vi "test_MultipleSessionsReserved_CallCreateSession_NothingAddedToConnectionMap.vi"(8 "error in":errorcluster) -> (0 "error out":errorcluster, 2 "result":string, 3 "pass":bool)   [LabVIEW 2020, in "MeasurementServerTests.lvlib"]
uses:
  MeasurementServerTests.lvlib
  Runtime/MeasurementLink Session Management/Session Reservation/Connection with Session.ctl
  Runtime/MeasurementLink Session Management/Session Reservation/Connection.ctl
  1a7c149c-48bc-4238-8756-811e337da54d.vi
  a956f7ee-c7e9-4639-884c-f4265dae6ecf.vi
  da202071-85ff-4e27-b7cd-0a9c854c86e4.vi
  da202071-85ff-4e27-b7cd-0a9c854c86e4.vi/7fd45821-cfd3-468e-85e7-fb0eb05eda95.vi
  Helpers/Fake Instrument/Fake Instrument.lvclass
  C:/dev/measurementlink-labview/Source/Runtime/MeasurementLink Instrument/IInstrument/IInstrument.lvclass
  Runtime/MeasurementLink Measurement Server/Helpers/Error Strings Global Internal.vi
  Runtime/MeasurementLink Session Management/Session Reservation/Create Sessions Dispatcher.vi
  Runtime/MeasurementLink Session Management/Session Reservation/Get Connections Dispatcher.vi
  Runtime/MeasurementLink Session Management/Session Reservation/Session Reservation.lvclass
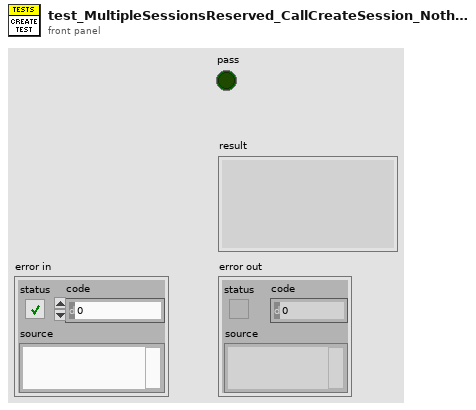
[diagram p1: front panel]
types:
  T1 = typedef "MeasurementLink Session Management.lvlib/Session Reservation.lvclass/Connection with Session.ctl" = cluster{"connection":T2, "session":variant}
  T2 = typedef "MeasurementLink Session Management.lvlib/Session Reservation.lvclass/Connection.ctl" = cluster{"pin or relay name":string, "site":i32, "instrument type id":string, "channel":string}
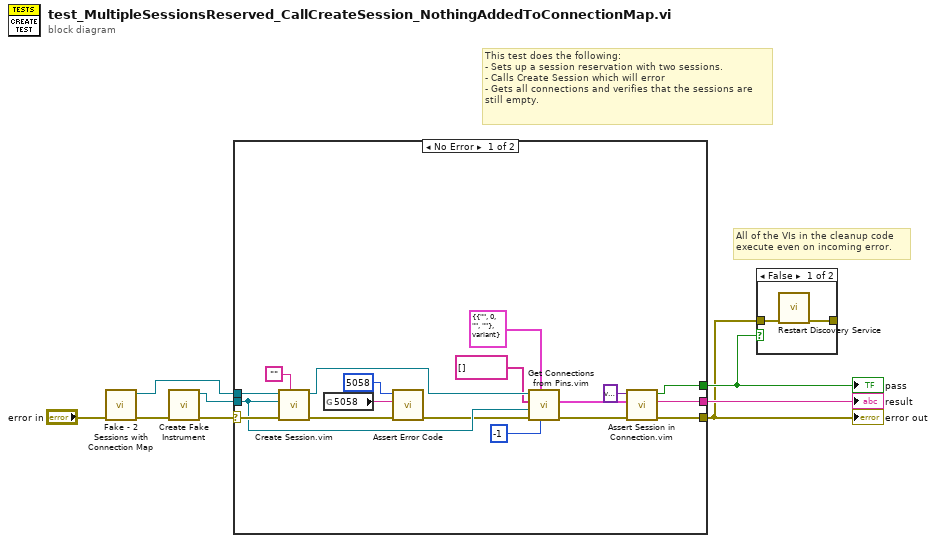
[diagram p0: block diagram]
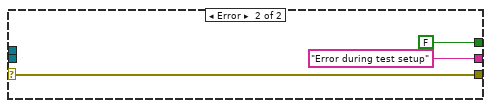
[diagram p2: hidden frame]
diagram:
  # "All of the VIs in the cleanup code\nexecute even on incoming error."
  # "This test does the following:\n- Sets up a session reservation with two sessions.\n- Calls Create Session which will error \n- Gets all connections and verifies that the sessions are\nstill empty."
  n1 = call "Fake - 2 Sessions with Connection Map.vi"("error in"="error in") -> ("error out"=w2:errorcluster, "session reservation out"=w1:refnum<class "Session Reservation.lvclass">)  [unwired: 9 in]
  n2 = call "Create Fake Instrument.vi"("error in"=w2) -> ("error out"=w5:errorcluster, "fake instrument out"=w4:refnum<class "Fake Instrument.lvclass">)  [unwired: 9 in]
  n3 = case shown="No Error" w5 {
    selector: w5 -> [w24 w26]
    tunnel: [w17 w26] -> w6
    tunnel: [w10 FALSE] -> w7
    tunnel: [w9 "Error during test setup" ("f")] -> w8
    tunnel: w4 -> [w20 _]
    tunnel: w1 -> [w25 _]
    frame No Error {
      n4 = call "Create Session.vim"("session type"="", "error in"=w24, "instrument"=w20, "session reservation in"=w25) -> ("error out"=w16:errorcluster, "session reservation out"=w22:refnum<class "Session Reservation.lvclass">)  [unwired: 4 in, 2 out]
      n5 = global read "Error Strings Global Internal.vi" "5058"() -> (w14:string)
      n6 = call "Assert Error Code.vi"("error in"=w16, "expected error description"=w14, "expected error code"=5058) -> ("error out"=w15:errorcluster)  [unwired: 6 in, 2 out]
      n7 = call "Get Connections from Pins.vim"("site"=-1, "connection type"=T1 {"connection"={"pin or relay name"="", "site"=0, "instrument type id"="", "channel"=""}, "session"=variant}, "error in"=w15, "instrument"=w20, "pin or relay names"=string[] [], "session reservation in"=w22) -> ("error out"=w17:errorcluster, "connections"=w12:T1[])  [unwired: 3 in, 1 out]
      n8 = call "Assert Session in Connection.vim"("actual connections"=w12, "expected session"=variant) -> ("result"=w9:string, "pass"=w10:bool)  [unwired: 8 in]
    }
    frame Error {
    }
  }
  "error out" <- w6
  "pass" <- w7
  "result" <- w8
  n9 = case shown="False" w7 {
    tunnel: w6 -> [w30 _]
    tunnel: [w29 _] -> _
    frame False {
      n10 = call "Restart Discovery Service.vi"("error in"=w30) -> ("error out"=w29:errorcluster)  [unwired: 10 in]
    }
    frame True {
    }
  }
